vi "Tear Down.vi"(8 "error in (no error)":errorcluster, 11 "Car Wash Display in":refnum<class "Car Wash Display.lvclass">) -> (0 "error out":errorcluster, 3 "Car Wash Display out":refnum<class "Car Wash Display.lvclass">)   [LabVIEW 2016, in "CLD Exam - Car Wash.lvlib" / "Car Wash Display.lvclass"]
uses:
  Car Wash Display.lvclass
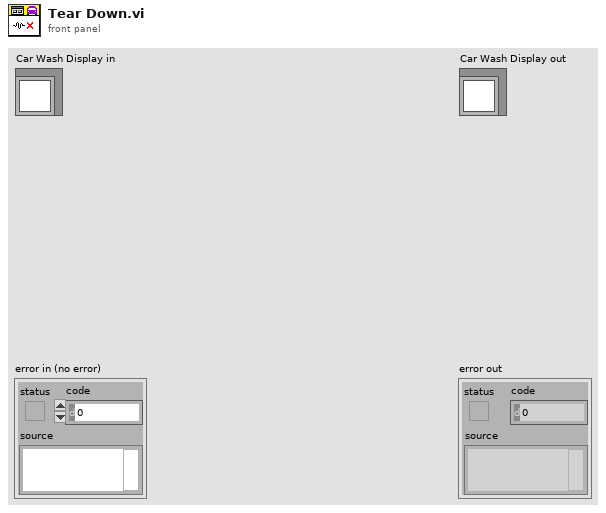
[diagram p1: front panel]
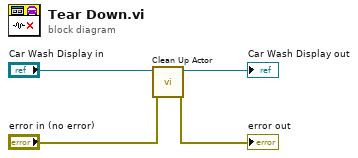
[diagram p0: block diagram]
diagram:
  n1 = call-dynamic "Clean Up Actor.vi"("error in (no error)"="error in (no error)", "Car Wash Console in"="Car Wash Display in") -> ("error out"=→"error out":errorcluster, "Car Wash Console out"=→"Car Wash Display out":refnum<class "Car Wash Display.lvclass">)  [unwired: 8 in]
